vi "Add Objects.vi"(8 "error in":errorcluster, 10 "elements":refnum<class>[](array[class]), 11 "Buffer in":refnum<data-value>) -> (0 "error out":errorcluster, 3 "Buffer":refnum<data-value>)   [LabVIEW 2013, in "ObjectBuffer.lvclass"]
doc: "This VI allows to input an array into the buffer. The location in the buffer is updated automatically.\n\nIf the input array is larger than the buffer then just take last elements of the input array and save them in the buffer. Also give a warning that this happened."
uses:
  ObjectBuffer.lvclass
  VariantBuffer/VariantBuffer.lvclass
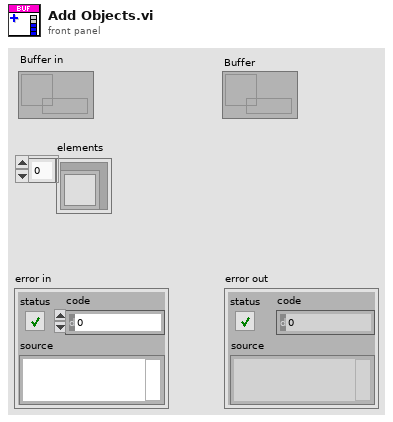
[diagram p1: front panel]
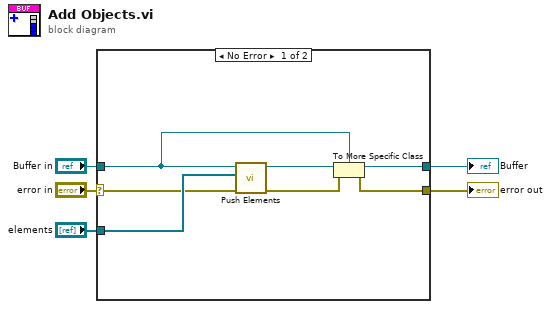
[diagram p0: block diagram]
diagram:
  n1 = case shown="No Error" "error in" {
    selector: "error in" -> [w8 w14]
    tunnel: "Buffer in" -> [w10 w13]
    tunnel: [w6 w13] -> w4
    tunnel: [w7 w14] -> w3
    tunnel: "elements" -> [w9 _]
    frame No Error {
      n2 = call "Push Elements.vi"("error in"=w8, "elements"=w9, "Buffer in"=w10) -> ("error out"=w11:errorcluster, "Buffer"=w12:refnum<data-value>)  [unwired: 7 in]
      n3 = To More Specific Class(target class=w10, reference=w12, error in=w11) -> (specific class reference=w6:refnum<data-value>, error out=w7:errorcluster)
    }
    frame Error {
    }
  }
  "error out" <- w3
  "Buffer" <- w4
